vi "CF,Oct to Fmin,Fmax.vi"(8 "BW":dbl, 10 "CF":dbl) -> (0 "Fmax":dbl, 2 "Fmin":dbl)   [LabVIEW 2020]
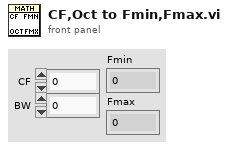
[diagram p1: front panel]
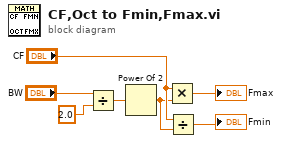
[diagram p0: block diagram]
diagram:
  n1 = Divide(x="BW", y=2.0) -> (x/y=w5:dbl)
  n2 = Power Of 2(x=w5) -> (2^x=w2:dbl)
  n3 = Multiply(x="CF", y=w2) -> (x*y=→"Fmax":dbl)
  n4 = Divide(x="CF", y=w2) -> (x/y=→"Fmin":dbl)
